vi "NanotecSMCPDDriver.default instrument setup.vi"(0 "VISA resource name":refnum<visa-resource-name>, 1 "contollerID":i32=-1, 5 "error in (no error)":errorcluster) -> (14 "VISA resource name out":refnum<visa-resource-name>, 15 "contollerID out":i32=-1, 19 "error out":errorcluster)   [LabVIEW 2014, in "NanotecSMCPDDriver.lvlib"]
doc: "This Utility VI sends a default command string to the instrument whenever a new VISA session is opened, or the instrument is reset. Use this VI as a subVI for the Initialize and Reset VIs. Altering this VI could cause these two VIs to operate incorrectly."
uses:
  NanotecSMCPDDriver.lvlib
  NanotecSMCPDDriver.positioning mode types.ctl
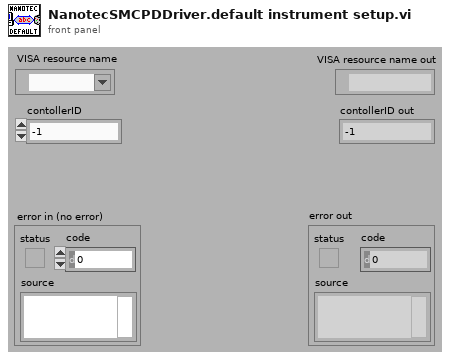
[diagram p1: front panel]
types:
  T1 = typedef "NanotecSMCPDDriver.lvlib/NanotecSMCPDDriver.positioning mode types.ctl" = enum16{"unknown", "relative positioning", "absolute positioning", "internal referencing", "external referencing"}
  T2 = typedef "NanotecSMCPDDriver.lvlib/NanotecSMCPDDriver.hardware types.ctl" = enum16{"unknown", "PD4", "PD4Ic", "PD2Ic", "SMCI32", "SMCI47"}
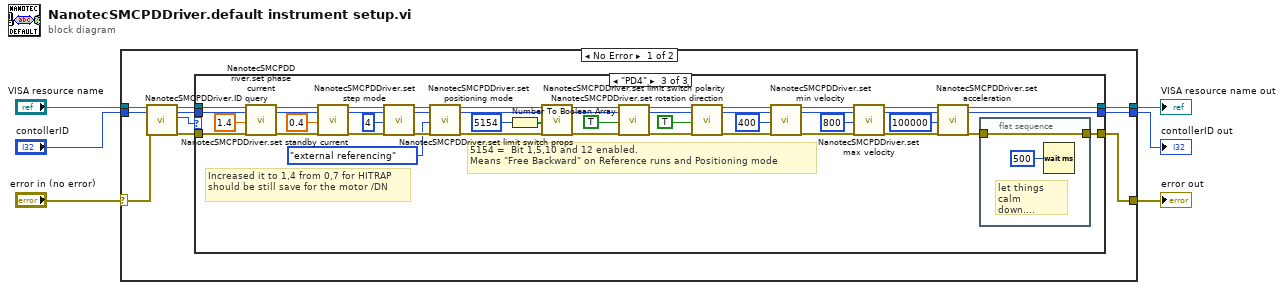
[diagram p0: block diagram]
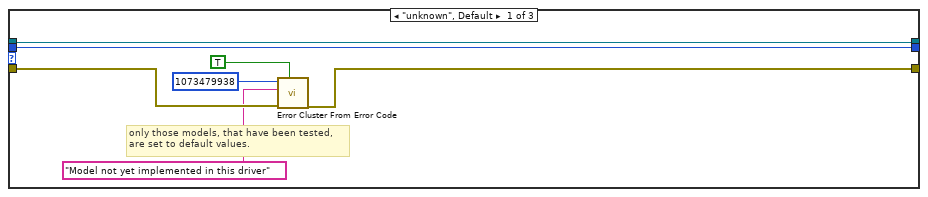
[diagram p2: hidden frame]
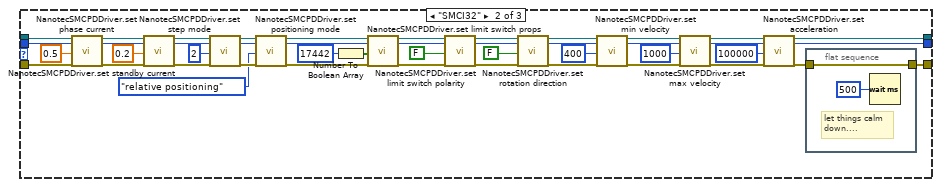
[diagram p3: hidden frame]
diagram:
  n1 = case shown="No Error" "error in (no error)" {
    selector: "error in (no error)" -> [w14 w120]
    tunnel: "VISA resource name" -> [w16 w119]
    tunnel: "contollerID" -> [w15 w118]
    tunnel: [w9 w120] -> w3
    tunnel: [w8 w119] -> w2
    tunnel: [w7 w118] -> w1
    frame No Error {
      n2 = call "NanotecSMCPDDriver.ID query.vi"("VISA resource name"=w16, "contollerID"=w15, "error in (no error)"=w14) -> ("VISA resource name out"=w11:refnum<visa-resource-name>, "contollerID out"=w10:i32, "hardwareType"=w13:T2, "error out"=w12:errorcluster)  [unwired: 13 out]
      n3 = case shown="\"PD4\"" w13 {
        tunnel: w12 -> [w23 w66 w113]
        tunnel: [w20 w25 w72] -> w8
        tunnel: w11 -> [w20 w68 w115]
        tunnel: [w19 w26 w73] -> w7
        tunnel: w10 -> [w19 w67 w114]
        tunnel: [w18 w43 w90] -> w9
        frame "unknown", Default {
          # "only those models, that have been tested,\nare set to default values."
          n4 = call <vilib>:"Error Cluster From Error Code.vi"("show call chain? (False)"=TRUE, "error in (no error)"=w23, "error message (\"\")"="Model not yet implemented in this driver" ("error message (\"\")"), "error code (0)"=1073479938) -> ("error out"=w18:errorcluster)  [unwired: 5 out]
        }
        frame "SMCI32" {
          n5 = call "NanotecSMCPDDriver.set phase current.vi"("VISA resource name"=w68, "contollerID"=w67, "phaseCurrent [A]"=0.5, "error in (no error)"=w66) -> ("VISA resource name out"=w64:refnum<visa-resource-name>, "contollerID out"=w63:i32, "error out"=w62:errorcluster)  [unwired: 13 out]
          n6 = call "NanotecSMCPDDriver.set standby current.vi"("VISA resource name"=w64, "contollerID"=w63, "standbyCurrent [A]"=0.2, "error in (no error)"=w62) -> ("VISA resource name out"=w60:refnum<visa-resource-name>, "contollerID out"=w59:i32, "error out"=w58:errorcluster)  [unwired: 13 out]
          n7 = call "NanotecSMCPDDriver.set step mode.vi"("VISA resource name"=w60, "contollerID"=w59, "stepMode"=2, "error in (no error)"=w58) -> ("VISA resource name out"=w50:refnum<visa-resource-name>, "contollerID out"=w48:i32, "error out"=w49:errorcluster)  [unwired: 13 out]
          n8 = call "NanotecSMCPDDriver.set positioning mode.vi"("VISA resource name"=w50, "contollerID"=w48, "positioningMode"=NanotecSMCPDDriver.positioning_mode_types."relative positioning", "error in (no error)"=w49) -> ("VISA resource name out"=w47:refnum<visa-resource-name>, "contollerID out"=w45:i32, "error out"=w46:errorcluster)  [unwired: 13 out]
          n9 = Number To Boolean Array(number=u16 17442) -> (Boolean array=w55:bool[])
          n10 = call "NanotecSMCPDDriver.set limit switch props.vi"("VISA resource name"=w47, "contollerID"=w45, "limitSwitchProperties (17442)"=w55, "error in (no error)"=w46) -> ("VISA resource name out"=w54:refnum<visa-resource-name>, "contollerID out"=w53:i32, "error out"=w52:errorcluster)  [unwired: 13 out]
          n11 = call "NanotecSMCPDDriver.set limit switch polarity.vi"("VISA resource name"=w54, "contollerID"=w53, "normallyClosed"=FALSE, "error in (no error)"=w52) -> ("VISA resource name out"=w40:refnum<visa-resource-name>, "contollerID out"=w41:i32, "error out"=w42:errorcluster)  [unwired: 13 out]
          n12 = call "NanotecSMCPDDriver.set rotation direction.vi"("VISA resource name"=w40, "contollerID"=w41, "clock-wise"=FALSE, "error in (no error)"=w42) -> ("VISA resource name out"=w38:refnum<visa-resource-name>, "contollerID out"=w37:i32, "error out"=w36:errorcluster)  [unwired: 13 out]
          n13 = call "NanotecSMCPDDriver.set min velocity.vi"("VISA resource name"=w38, "contollerID"=w37, "minVelocity [Hz]"=400, "error in (no error)"=w36) -> ("VISA resource name out"=w35:refnum<visa-resource-name>, "contollerID out"=w34:i32, "error out"=w33:errorcluster)  [unwired: 13 out]
          n14 = call "NanotecSMCPDDriver.set max velocity.vi"("VISA resource name"=w35, "contollerID"=w34, "maxVelocity [Hz]"=1000, "error in (no error)"=w33) -> ("VISA resource name out"=w30:refnum<visa-resource-name>, "contollerID out"=w29:i32, "error out"=w28:errorcluster)  [unwired: 13 out]
          n15 = call "NanotecSMCPDDriver.set acceleration.vi"("VISA resource name"=w30, "contollerID"=w29, "acceleration [Hz/s]"=100000, "error in (no error)"=w28) -> ("VISA resource name out"=w25:refnum<visa-resource-name>, "contollerID out"=w26:i32, "error out"=w27:errorcluster)  [unwired: 13 out]
          n16 = flat-sequence {
            tunnel: w27 -> [w70]
            tunnel: [w70] -> w43
            frame #0 {
              # "let things calm\ndown...."
              n17 = Wait (ms)(milliseconds to wait=u32 500) -> ()  [unwired: 1 out]
            }
          }
        }
        frame "PD4" {
          # "Increased it to 1,4 from 0,7 for HITRAP  \nshould be still save for the motor /DN"
          # "5154 =  Bit 1,5,10 and 12 enabled.\nMeans \"Free Backward\" on Reference runs and Positioning mode"
          n18 = call "NanotecSMCPDDriver.set phase current.vi"("VISA resource name"=w115, "contollerID"=w114, "phaseCurrent [A]"=1.4, "error in (no error)"=w113) -> ("VISA resource name out"=w111:refnum<visa-resource-name>, "contollerID out"=w110:i32, "error out"=w109:errorcluster)  [unwired: 13 out]
          n19 = call "NanotecSMCPDDriver.set standby current.vi"("VISA resource name"=w111, "contollerID"=w110, "standbyCurrent [A]"=0.4, "error in (no error)"=w109) -> ("VISA resource name out"=w107:refnum<visa-resource-name>, "contollerID out"=w106:i32, "error out"=w105:errorcluster)  [unwired: 13 out]
          n20 = call "NanotecSMCPDDriver.set step mode.vi"("VISA resource name"=w107, "contollerID"=w106, "stepMode"=4, "error in (no error)"=w105) -> ("VISA resource name out"=w97:refnum<visa-resource-name>, "contollerID out"=w95:i32, "error out"=w96:errorcluster)  [unwired: 13 out]
          n21 = call "NanotecSMCPDDriver.set positioning mode.vi"("VISA resource name"=w97, "contollerID"=w95, "positioningMode"=NanotecSMCPDDriver.positioning_mode_types."external referencing", "error in (no error)"=w96) -> ("VISA resource name out"=w94:refnum<visa-resource-name>, "contollerID out"=w92:i32, "error out"=w93:errorcluster)  [unwired: 13 out]
          n22 = Number To Boolean Array(number=u16 5154) -> (Boolean array=w102:bool[])
          n23 = call "NanotecSMCPDDriver.set limit switch props.vi"("VISA resource name"=w94, "contollerID"=w92, "limitSwitchProperties (17442)"=w102, "error in (no error)"=w93) -> ("VISA resource name out"=w101:refnum<visa-resource-name>, "contollerID out"=w100:i32, "error out"=w99:errorcluster)  [unwired: 13 out]
          n24 = call "NanotecSMCPDDriver.set limit switch polarity.vi"("VISA resource name"=w101, "contollerID"=w100, "normallyClosed"=TRUE, "error in (no error)"=w99) -> ("VISA resource name out"=w87:refnum<visa-resource-name>, "contollerID out"=w88:i32, "error out"=w89:errorcluster)  [unwired: 13 out]
          n25 = call "NanotecSMCPDDriver.set rotation direction.vi"("VISA resource name"=w87, "contollerID"=w88, "clock-wise"=TRUE, "error in (no error)"=w89) -> ("VISA resource name out"=w85:refnum<visa-resource-name>, "contollerID out"=w84:i32, "error out"=w83:errorcluster)  [unwired: 13 out]
          n26 = call "NanotecSMCPDDriver.set min velocity.vi"("VISA resource name"=w85, "contollerID"=w84, "minVelocity [Hz]"=400, "error in (no error)"=w83) -> ("VISA resource name out"=w82:refnum<visa-resource-name>, "contollerID out"=w81:i32, "error out"=w80:errorcluster)  [unwired: 13 out]
          n27 = call "NanotecSMCPDDriver.set max velocity.vi"("VISA resource name"=w82, "contollerID"=w81, "maxVelocity [Hz]"=800, "error in (no error)"=w80) -> ("VISA resource name out"=w77:refnum<visa-resource-name>, "contollerID out"=w76:i32, "error out"=w75:errorcluster)  [unwired: 13 out]
          n28 = call "NanotecSMCPDDriver.set acceleration.vi"("VISA resource name"=w77, "contollerID"=w76, "acceleration [Hz/s]"=100000, "error in (no error)"=w75) -> ("VISA resource name out"=w72:refnum<visa-resource-name>, "contollerID out"=w73:i32, "error out"=w74:errorcluster)  [unwired: 13 out]
          n29 = flat-sequence {
            tunnel: w74 -> [w117]
            tunnel: [w117] -> w90
            frame #0 {
              # "let things calm\ndown...."
              n30 = Wait (ms)(milliseconds to wait=u32 500) -> ()  [unwired: 1 out]
            }
          }
        }
      }
    }
    frame Error {
    }
  }
  "error out" <- w3
  "VISA resource name out" <- w2
  "contollerID out" <- w1
